vi "Timer_StateMachine_Complex_Example.vi"() -> ()   [LabVIEW 2019]
uses:
  <vilib>/Utility/semaphor.llb/Obtain Semaphore Reference.vi
  <vilib>/Rock Robotics/WPI/ThirdParty/JAS_Junk/TrajLib/Trajectory_Library.lvlib
panel:
  out "State":i32
  in  "Tab Control":enum32{"Control Panel"}(tab)
  in  "Start Sequence":bool
  out "Trend":cluster{"CurrentTImer":dbl, "CurrentTImer":dbl}(graph)
  out "Action 1":bool
  out "Timer 2":dbl
  out "Timer 1":dbl
  in  "Stop Timer":bool
  out "Action 2":bool
  # "Timer - State Machine - Example"
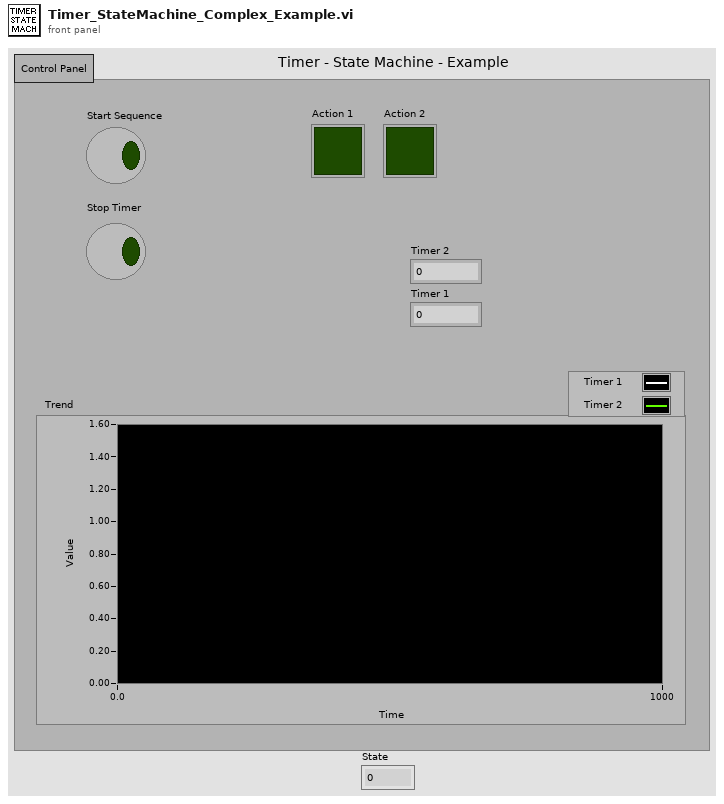
[diagram p1: front panel]
types:
  T1 = typedef "Trajectory_Library.lvlib/TIMER.ctl" = cluster{"StartTime":dbl, "Accumulated TIme":dbl, "Running":bool, "semaphore":T2}
  T2 = typedef "Semaphore RefNum" = refnum<k1>
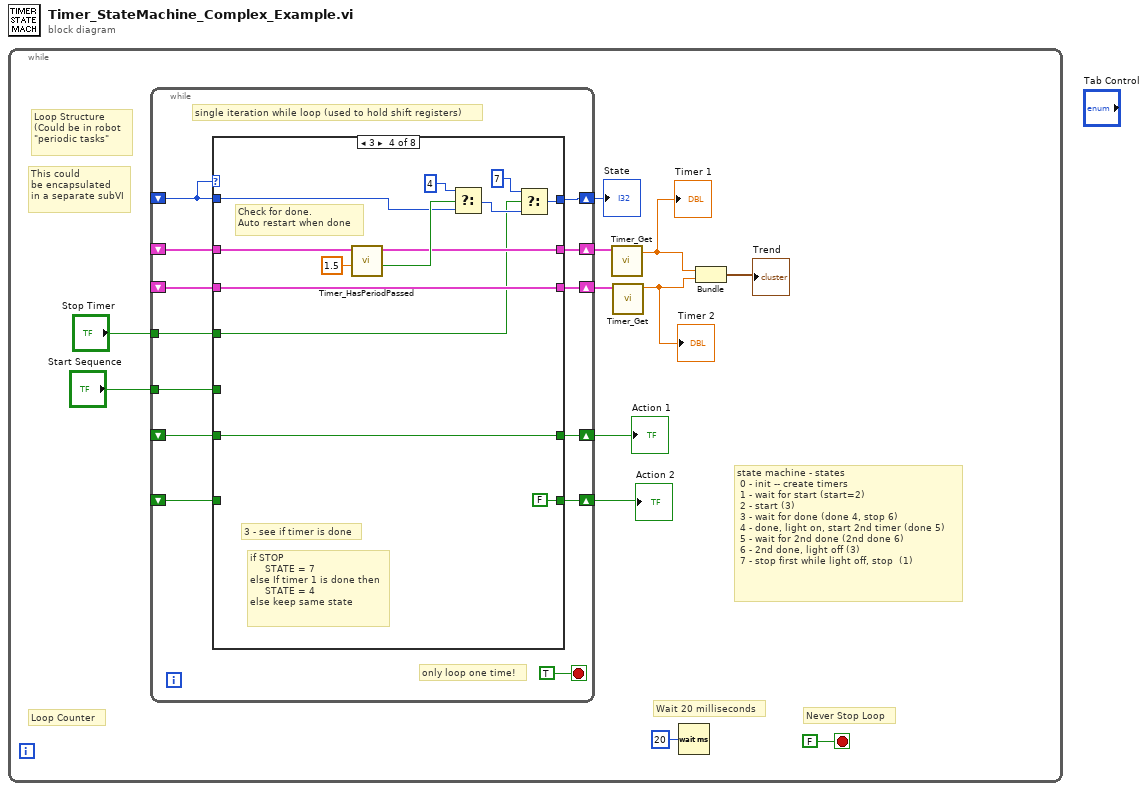
[diagram p0: block diagram]
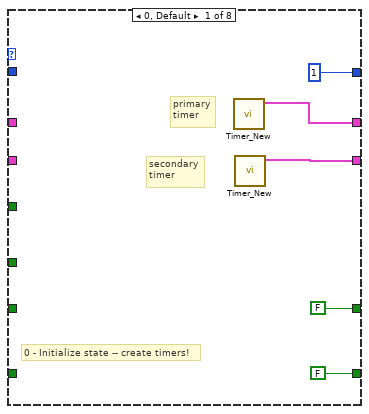
[diagram p2: hidden frame]
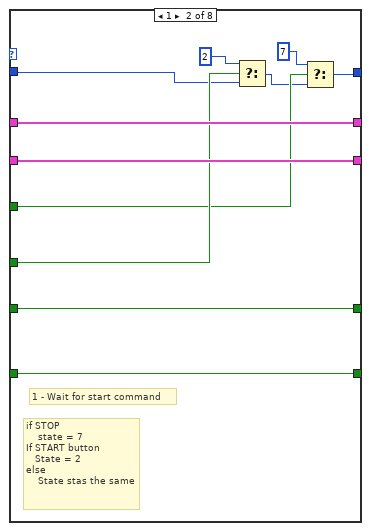
[diagram p3: hidden frame]
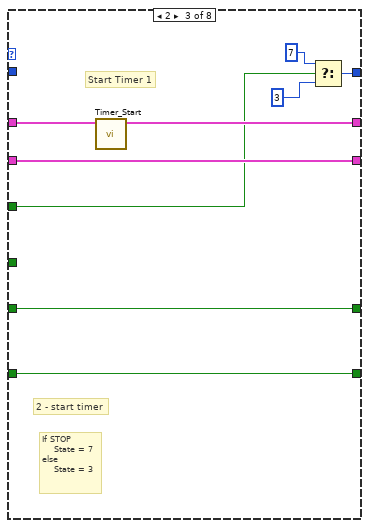
[diagram p4: hidden frame]
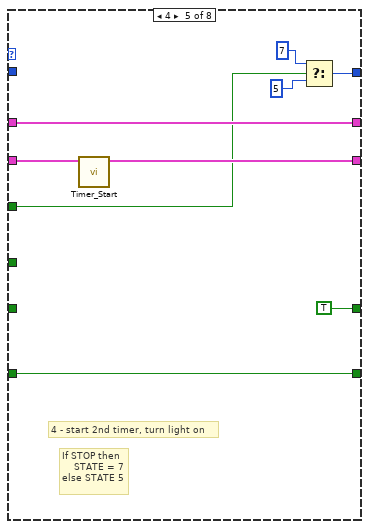
[diagram p5: hidden frame]
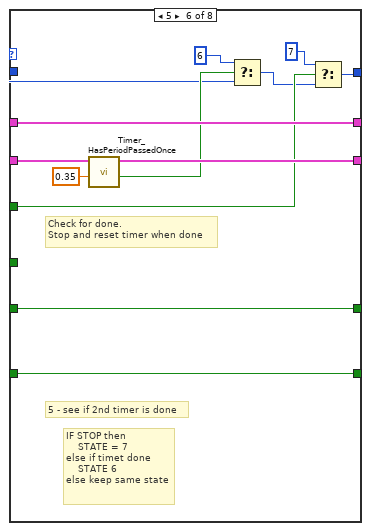
[diagram p6: hidden frame]
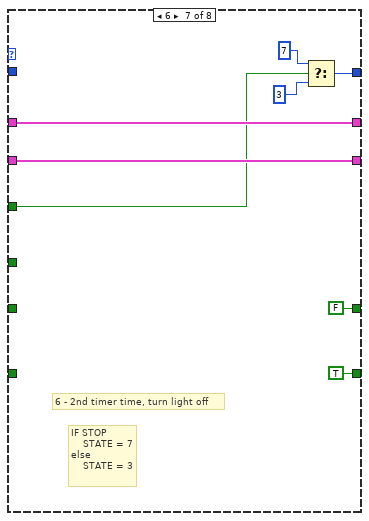
[diagram p7: hidden frame]
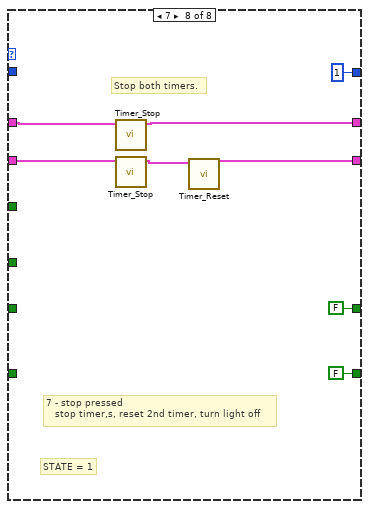
[diagram p8: hidden frame]
diagram:
  n1 = while {
    stop <- FALSE stop-if-true
    # "This could\nbe encapsulated\nin a separate subVI"
    # "Loop Structure\n(Could be in robot\n\"periodic tasks\""
    # "state machine - states\n 0 - init -- create timers\n 1 - wait for start (start=2)\n 2 - start (3)\n 3 - wait for done (done 4, stop 6)\n 4 - done, light on, start 2nd timer (done 5)\n 5 - wait for 2nd done (2nd done 6)\n 6 - 2nd done, light off (3)\n 7 - stop first while light off, stop  (1)"
    # "Loop Counter"
    # "Never Stop Loop"
    # "Wait 20 milliseconds"
    n2 = while {
      shift-right: [w22] -> w10
      shift-left: _ -> [w20]
      shift-right: [w24] -> w7
      shift-left: _ -> [w19]
      shift-right: [w23] -> w6
      shift-left: _ -> [w18]
      tunnel: "Start Sequence" -> [w21]
      shift-right: [w17] -> w8
      shift-left: _ -> [w16]
      tunnel: "Stop Timer" -> [w15]
      shift-right: [w14] -> w1
      shift-left: _ -> [w13]
      stop <- TRUE stop-if-true
      # "only loop one time!"
      # "single iteration while loop (used to hold shift registers)"
      n3 = case shown="3" w20 {
        tunnel: [w30 w41 w49 w59 w72 w85 w92 w96] -> w24
        tunnel: [w29 w40 w48 w57 w70 w81 w91 w97] -> w23
        tunnel: [1 w32 w43 w52 w67 w76 w88 1 ("t")] -> w22
        tunnel: w21 -> [_ w39 _ _ _ _ _ _]
        tunnel: w20 -> [_ w38 _ w58 _ w78 _ _]
        tunnel: w19 -> [_ w41 w50 w60 w72 w85 w92 w100]
        tunnel: w18 -> [_ w40 w48 w57 w71 w82 w91 w99]
        tunnel: [FALSE w36 w47 w56 TRUE w84 FALSE FALSE] -> w17
        tunnel: w16 -> [_ w36 w47 w56 _ w84 _ _]
        tunnel: w15 -> [_ w34 w44 w53 w65 w75 w87 _]
        tunnel: [FALSE w31 w42 FALSE w64 w73 TRUE FALSE] -> w14
        tunnel: w13 -> [_ w31 w42 _ w64 w73 _ _]
        frame 0, Default {
          # "0 - Initialize state -- create timers!"
          # "secondary\ntimer"
          # "primary\ntimer"
          n4 = call <vilib>:"Timer_New.vi"() -> ("TIMER"=w30:T1)  [unwired: 11 in]
          n5 = call <vilib>:"Timer_New.vi"() -> ("TIMER"=w29:T1)  [unwired: 11 in]
        }
        frame 1 {
          # "if STOP \n    state = 7\nIf START button\n   State = 2\nelse\n    State stas the same"
          # "1 - Wait for start command"
          n6 = Select(t=2, s=w39, f=w38) -> (s? t:f=w33:i32)
          n7 = Select(t=7, s=w34, f=w33) -> (s? t:f=w32:i32)
        }
        frame 2 {
          # "If STOP\n    State = 7\nelse\n    State = 3"
          # "Start Timer 1"
          # "2 - start timer"
          n8 = call <vilib>:"Timer_Start.vi"("in Timer"=w50) -> ("out Timer"=w49:T1)  [unwired: 10 in]
          n9 = Select(t=7, s=w44, f=3) -> (s? t:f=w43:i32)
        }
        frame 3 {
          # "if STOP \n     STATE = 7\nelse If timer 1 is done then\n     STATE = 4\nelse keep same state"
          # "Check for done.\nAuto restart when done"
          # "3 - see if timer is done"
          n10 = call <vilib>:"Timer_HasPeriodPassed.vi"("Period"=1.5, "in Timer"=w60) -> ("Expired"=w61:bool, "out Timer"=w59:T1)  [unwired: 7 in, 1 out]
          n11 = Select(t=4, s=w61, f=w58) -> (s? t:f=w54:i32)
          n12 = Select(t=7, s=w53, f=w54) -> (s? t:f=w52:i32)
        }
        frame 4 {
          # "If STOP then\n    STATE = 7\nelse STATE 5"
          # "4 - start 2nd timer, turn light on"
          n13 = call <vilib>:"Timer_Start.vi"("in Timer"=w71) -> ("out Timer"=w70:T1)  [unwired: 10 in]
          n14 = Select(t=7, s=w65, f=5 ("t")) -> (s? t:f=w67:i32)
        }
        frame 5 {
          # "IF STOP then\n    STATE = 7\nelse if timet done\n    STATE 6\nelse keep same state"
          # "Check for done.\nStop and reset timer when done"
          # "5 - see if 2nd timer is done"
          n15 = call <vilib>:"Timer_HasPeriodPassedOnce.vi"("Period"=0.35, "in Timer"=w82) -> ("Expired"=w79:bool, "out Timer"=w81:T1)  [unwired: 7 in, 1 out]
          n16 = Select(t=6, s=w79, f=w78) -> (s? t:f=w74:i32)
          n17 = Select(t=7, s=w75, f=w74) -> (s? t:f=w76:i32)
        }
        frame 6 {
          # "IF STOP\n    STATE = 7\nelse\n    STATE = 3"
          # "6 - 2nd timer time, turn light off"
          n18 = Select(t=7, s=w87, f=3 ("t")) -> (s? t:f=w88:i32)
        }
        frame 7 {
          # "STATE = 1"
          # "Stop both timers."
          # "7 - stop pressed\n   stop timer,s, reset 2nd timer, turn light off"
          n19 = call <vilib>:"Timer_Stop.vi"("in Timer"=w100) -> ("out Timer"=w96:T1)  [unwired: 10 in]
          n20 = call <vilib>:"Timer_Stop.vi"("in Timer"=w99) -> ("out Timer"=w98:T1)  [unwired: 10 in]
          n21 = call <vilib>:"Timer_Reset.vi"("in TIMER"=w98) -> ("out TIMER"=w97:T1)  [unwired: 10 in]
        }
      }
    }
    "Action 1" <- w8
    "State" <- w10
    "Action 2" <- w1
    n22 = call <vilib>:"Timer_Get.vi"("TIMER"=w7) -> ("CurrentTImer"=w5:dbl)  [unwired: 10 in]
    "Timer 1" <- w5
    n23 = call <vilib>:"Timer_Get.vi"("TIMER"=w6) -> ("CurrentTImer"=w4:dbl)  [unwired: 10 in]
    "Timer 2" <- w4
    n24 = Wait (ms)(milliseconds to wait=u32 20) -> ()  [unwired: 1 out]
    n25 = Bundle("CurrentTImer"=w5, "CurrentTImer"=w4) -> (→"Trend":cluster{"CurrentTImer":dbl, "CurrentTImer":dbl})  [unwired: 1 in]
  }
